vi "poly_unpack_controls_page.vi"(2 "recursivelly? (T)":bool=TRUE, 7 "ctrl ref":refnum<vi>) -> (8 "ctrls in pages":refnum<vi>[](array[refnum]))   [LabVIEW 2015]
uses:
  poly_is_specific_control_PageSelector.vi
  cores/core_is_specific_controll.vi
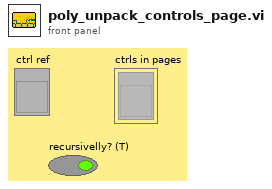
[diagram p1: front panel]
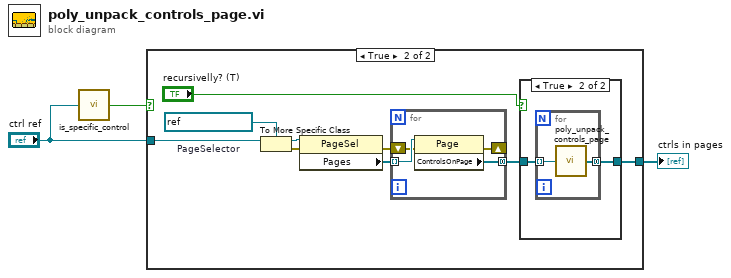
[diagram p0: block diagram]
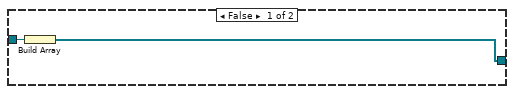
[diagram p2: hidden frame]
diagram:
  n1 = call-poly "is_specific_control.vi"("ctrl ref"="ctrl ref") -> ("is PageSelector?"=w1:bool)  [unwired: 8 in]
  n2 = case shown="True" w1 {
    tunnel: [w4 w7] -> w3
    tunnel: "ctrl ref" -> [w5 w12]
    frame False {
      n3 = Build Array(w5) -> (w4:refnum<vi>[])
    }
    frame True {
      w13 = refnum<vi> refnum  # PageSelector
      n4 = To More Specific Class(target class=w13, reference=w12) -> (specific class reference=w11:refnum<vi>, error out=w10:errorcluster)  [unwired: 1 in]
      n5 = property class="PageSel"(reference=w11, error in=w10) -> (error out=w9:errorcluster, "Pages"=w14:refnum<vi>[])  [unwired: 1 out]
      n6 = for {
        tunnel: w14 -> [w23] mode=indexing
        tunnel: [w22] -> w8 mode=concatenating
        shift-right: [w20] -> _
        shift-left: w9 -> [w21]
        n7 = property class="Page"(reference=w23, error in=w21) -> (error out=w20:errorcluster, "ControlsOnPage"=w22:refnum<vi>[])  [unwired: 1 out]
      }
      n8 = case shown="True" "recursivelly? (T)" {
        tunnel: w8 -> [w15 w17]
        tunnel: [w15 w16] -> w7
        frame False {
        }
        frame True {
          n9 = for {
            tunnel: w17 -> [w19] mode=indexing
            tunnel: [w18] -> w16 mode=concatenating
            n10 = call "poly_unpack_controls_page.vi"("ctrl ref"=w19) -> ("ctrls in pages"=w18:refnum<vi>[])  [unwired: 14 in]
          }
        }
      }
    }
  }
  "ctrls in pages" <- w3
